vi "Show DB.vi"() -> ()   [LabVIEW 2017]
doc: "Shows the contents of the database."
uses:
  <vilib>/drjdpowell/SQLite Library/SQL Connection/Open (path).vi
  <vilib>/drjdpowell/SQLite Library/SQL Connection/Open (string).vi
  Common64/Database/SQ Lite/SQ Lite Globals.vi
  <vilib>/AdvancedString/Path To Command Line String.vi
  <vilib>/drjdpowell/SQLite Library/SQL Connection/Connection.lvclass
panel:
  out "error out":errorcluster
  out "Result Set":string[][](table) caption="Database Albums"
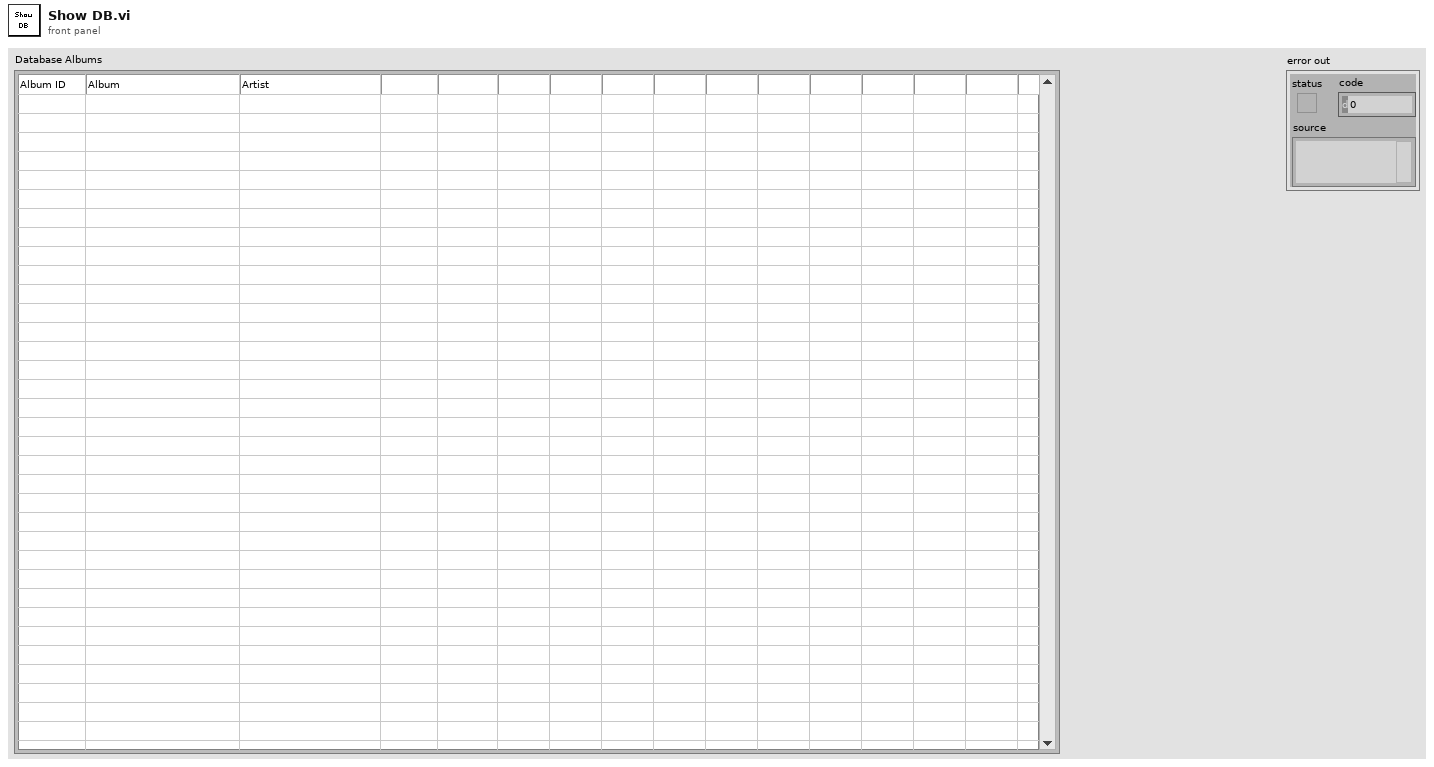
[diagram p1: front panel]
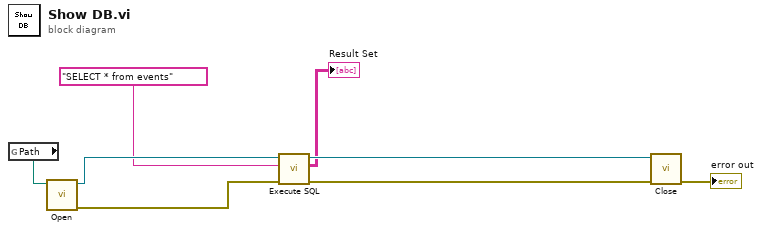
[diagram p0: block diagram]
diagram:
  n1 = global read "SQ Lite Globals.vi" "Path"() -> (w1:path)
  n2 = call-poly <vilib>:"Open.vi"("db file"=w1) -> ("error out"=w5:errorcluster, "SQLite Connection"=w6:refnum<class "Connection.lvclass">)  [unwired: 9 in]
  n3 = call <vilib>:"Execute SQL.vi"("error in (no error)"=w5, "SQL"="SELECT * from events", "SQLite Connection in"=w6) -> ("error out"=w7:errorcluster, "Result Set"=→"Result Set":string[][], "SQLite Connection"=w8:refnum<class "Connection.lvclass">)  [unwired: 5 in, 1 out]
  n4 = call-dynamic "Close.vi"("error in (no error)"=w7, "SQLite Connection in"=w8) -> ("error out"=→"error out":errorcluster)  [unwired: 9 in]
